vi "Get Nice Range.vi"(8 "Type":enum16{"Max", "Min"}(ring), 10 "Difference":sgl, 11 "Input":sgl) -> (3 "Output":sgl)   [LabVIEW 2017, in "3D Plot Datatype.lvclass"]
uses:
  <vilib>/Math Plots/3D Math Plots/3D Plot/3D Plot Datatype/3D Plot Datatype.lvclass
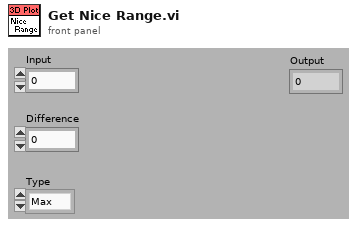
[diagram p1: front panel]
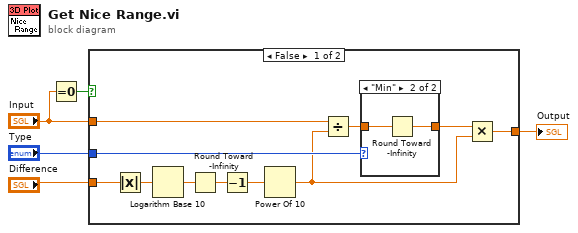
[diagram p0: block diagram]
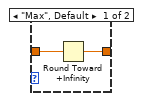
[diagram p2: hidden frame]
diagram:
  n1 = Equal To 0?(x="Input") -> (x = 0?=w4:bool)
  n2 = case shown="False" w4 {
    tunnel: "Input" -> [w8 w21]
    tunnel: [w12 w21] -> w3
    tunnel: "Type" -> [w16 _]
    tunnel: "Difference" -> [w11 _]
    frame False {
      n3 = Absolute Value(x=w11) -> (abs(x)=w10:sgl)
      n4 = Logarithm Base 10(1:w10) -> (0:w7:sgl)
      n5 = Round Toward -Infinity(1:w7) -> (0:w9:sgl)
      n6 = Decrement(x=w9) -> (x-1=w6:sgl)
      n7 = Power Of 10(x=w6) -> (10^x=w13:sgl)
      n8 = Divide(x=w8, y=w13) -> (x/y=w15:sgl)
      n9 = case shown="\"Min\"" w16 {
        tunnel: w15 -> [w18 w20]
        tunnel: [w17 w19] -> w14
        frame "Max", Default {
          n10 = Round Toward +Infinity(x=w18) -> (ceil(x): smallest int >= x=w17:sgl)
        }
        frame "Min" {
          n11 = Round Toward -Infinity(1:w20) -> (0:w19:sgl)
        }
      }
      n12 = Multiply(x=w14, y=w13) -> (x*y=w12:sgl)
    }
    frame True {
    }
  }
  "Output" <- w3
